vi "Insert Topic Actor by Name.vi"(8 "error in (no error)":errorcluster, 9 "Topic Actor Descriptor":refnum<class "Topic Actor Descriptor.lvclass">, 10 "Topic Actor":string, 11 "Topic Actor Look Up Table in":refnum<class "Topic Actor Look Up Table.lvclass">) -> (0 "error out":errorcluster, 2 "Replaced?":bool, 3 "Topic Actor Look Up Table out":refnum<class "Topic Actor Look Up Table.lvclass">)   [LabVIEW 2016, in "Stream Mediator.lvlib" / "Topic Actor Look Up Table.lvclass"]
doc: "--\nCopyright © 2017 Composed SystemsI All rights reserved.\n\nAuthor: Jon McBee <jon.mcbee@composed.io>\n\nThis library is provided \"AS IS\" ,WITHOUT WARRANTIES OR\nCONDITIONS OF ANY KIND, either express or implied.\n\nComposed Systems -- composed.io\n\nStream 0.0.1.1\nJon McBee - Composed Systems\nCopyright (c) 2017, Composed Systems"
uses:
  <userlib>/Composed Systems/Stream/Mediator/Classes/Topic Actor Look Up Table/Topic Actor Look Up Table.lvclass
  C:/Program Files (x86)/National Instruments/LabVIEW 2016/user.lib/Composed Systems/Stream/Look Up Table/Look Up Table/Look Up Table.lvclass
  <userlib>/Composed Systems/Stream/Mediator/Classes/Topic Actor Descriptor/Topic Actor Descriptor.lvclass
  <userlib>/Composed Systems/Stream/Look Up Table/Look Up Table/Look Up Table.lvclass
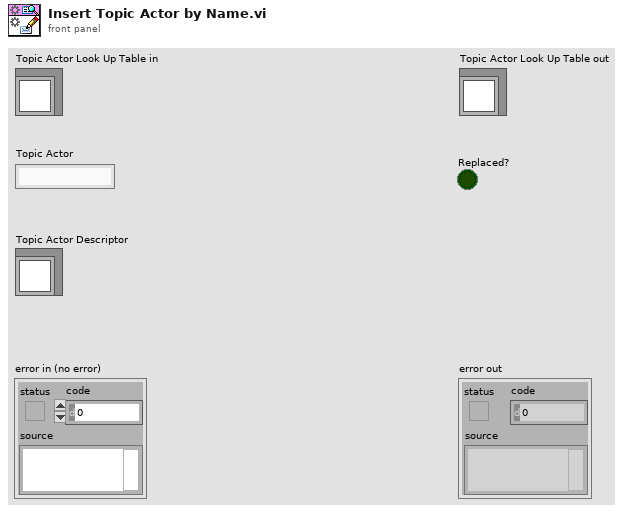
[diagram p1: front panel]
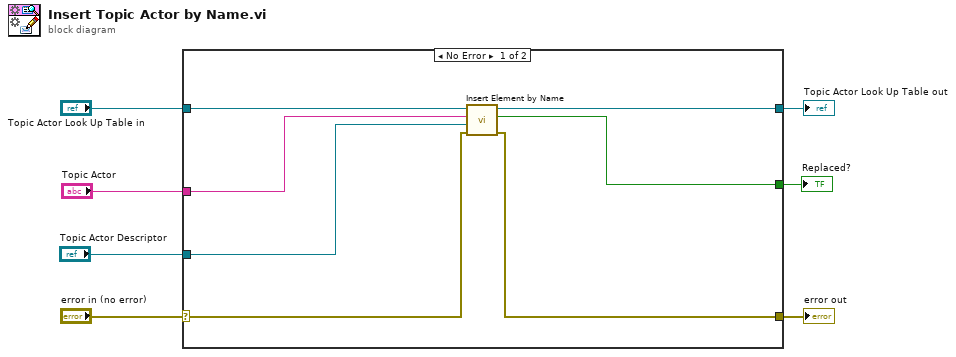
[diagram p0: block diagram]
diagram:
  n1 = case shown="No Error" "error in (no error)" {
    selector: "error in (no error)" -> [w14 w16]
    tunnel: [w13 w16] -> w6
    tunnel: [w11 w15] -> w4
    tunnel: "Topic Actor Look Up Table in" -> [w12 w15]
    tunnel: "Topic Actor" -> [w9 _]
    tunnel: "Topic Actor Descriptor" -> [w8 _]
    tunnel: [w10 _] -> w2
    frame No Error {
      n2 = call <userlib>:"Insert Element by Name.vi"("error in (no error)"=w14, "Variant"=w8, "Name"=w9, "Look Up Table in"=w12) -> ("error out"=w13:errorcluster, "Replaced?"=w10:bool, "Look Up Table out"=w11:refnum<class "Topic Actor Look Up Table.lvclass">)  [unwired: 5 in]
    }
    frame Error {
    }
  }
  "error out" <- w6
  "Topic Actor Look Up Table out" <- w4
  "Replaced?" <- w2
